vi "Write.vi"(8 "error in (no error)":errorcluster, 11 "TDMS_Writer in":refnum<class "TDMS_Writer.lvclass">) -> (0 "error out":errorcluster, 3 "TDMS_Writer out":refnum<class "TDMS_Writer.lvclass">)   [LabVIEW 2024, in "Data.lvlib" / "TDMS_Writer.lvclass"]
uses:
  TDMS_Writer.lvclass
  DataWriter/DataWriter.lvclass
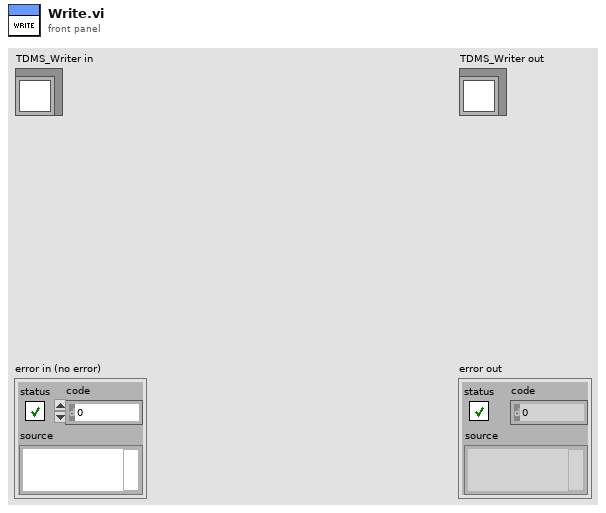
[diagram p1: front panel]
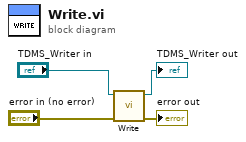
[diagram p0: block diagram]
diagram:
  n1 = call-parent "Write.vi"("error in (no error)"="error in (no error)", "DataWriter in"="TDMS_Writer in") -> ("error out"=→"error out":errorcluster, "DataWriter out"=→"TDMS_Writer out":refnum<class "TDMS_Writer.lvclass">)  [unwired: 8 in]
